vi "Expt4_MT PSK Transceiver_Student_lab.vi"(0 "Message Symbols":i32=1000, 5 "Eb/N0, dB":dbl(slide)=40.0 scale=0.0..80.0, 7 "TX Filter":T1(ring)=enum."Root Raised Cos", 9 "Reset":bool=TRUE, 14 "?":T2(tab)=enum."Constellation (RX output)") -> (3 "PSK System Parameters":T5={"samples per symbol (16)"=4, "symbol map"=[0.7071067811865476+0.7071067811865475i, -0.7071067811865475+0.7071067811865476i, 0.7071067811865474-0.7071067811865477i, -0.7071067811865477-0.7071067811865475i], "differential PSK"=enum."disable", "PSK type"=0} {"PSK type" items=["normal", "shifted", "offset"]; "symbol map" format="%.3f"}, 4 "Output Complex Waveform":cluster{"t0":dbl, "dt":dbl, "Values":cdb[]} {"Values" format="%.3f"; "dt" format="%^.2e"; "t0" format="%.4f"}, 6 "Transmitted  Bits":i8[](array[numeric]), 8 "Received Bits":i8[](array[numeric]), 10 "Bit Error Rate":dbl format="%.4e", 13 "Last Sync Found Index":dbl format="%.4f", 15 "Error Out":errorcluster)   [LabVIEW 2020]
doc: "This example demonstrates generation and analysis of PSK modulated signals. You can specify transmit filter parameters, Eb/No, and frequency offset. This example demonstrates programming techniques for resetting the transmitter in cases where the receiver (demodulator) lock is lost. You can see the results of the demodulation on an eye-diagram plot, and perform measurements such as bit error rate."
uses:
  <vilib>/addons/Modulation/niDMT.lvlib
  <vilib>/addons/Modulation/Digital/General/MT Format Eye Diagram (complex).vi
  <vilib>/addons/Modulation/niAMT.lvlib
  <vilib>/addons/Modulation/Digital/Support/Controls/PSK System Parameters.ctl
panel:
  out "Estimated Eb/N0(dB)":dbl
  out "Frequency Offset, Hz":dbl=0.0014081098665354938 format="%.2f"
  in  "Frequency Offset, Hz":dbl(slide) scale=-1000.0..1000.0
  in  "Symbol Rate":dbl=100000.0 step=1000.0 format="%.2p"
  in  "M-PSK":enum16{"2", "4", "8", "16", "32", "64"}(ring)=enum."4"
  out "Modulation Error Ratio, dB":dbl format="%.2f"
  out "BER Trigger Found":bool
  in  "Stop":bool
  out "TX Symbols":T3(graph)={{"1/x"=0.0, 1e-05, [], 1}, []}
  out "FFT Magnitude Spectrum":cluster{dbl, dbl, dbl[]}(graph)={-199899.99999999997, 99.99999999999999, []}
  out "Constellation graph":T4(graph)
  out "RX Symbols":T3(graph)={{"1/x"=0.0, 1e-05, [], 1}, []}
  in  "autoscale":bool
  out "Constellation Graph":T4(graph)
  in  "Display I/Q":enum16{"I", "Q"}(ring)=enum."Q"
  out "Eye Diagram":cluster{"t0":dbl, "dt":dbl, "Y":dbl[]}[](graph)
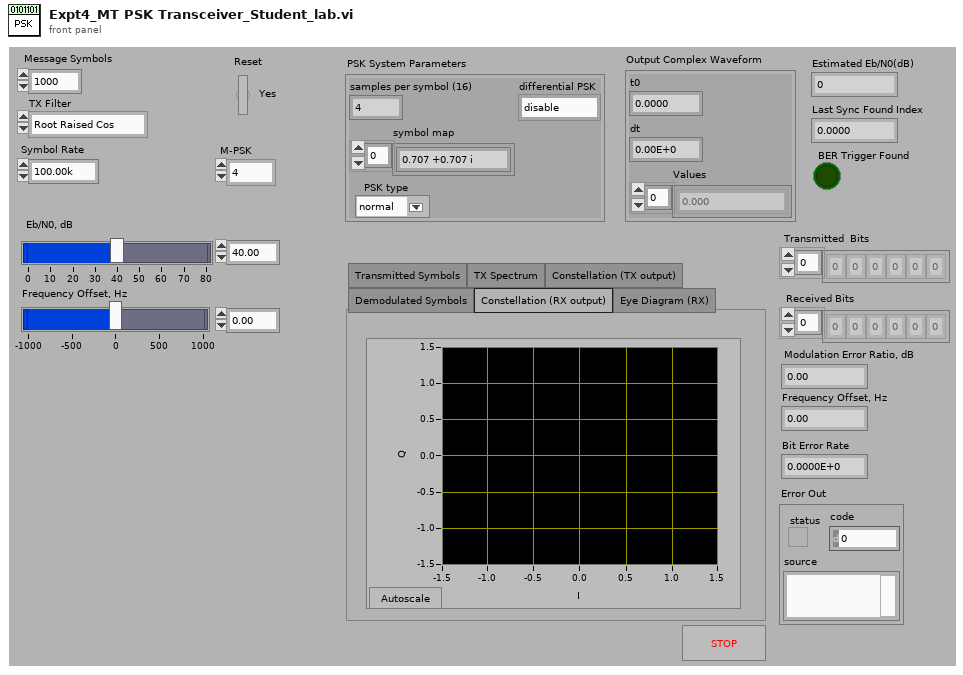
[diagram p1: front panel]
types:
  T1 = enum16{"none", "Raised Cosine", "Root Raised Cos", "Gaussian"}
  T2 = enum32{"Transmitted Symbols", "TX Spectrum", "Constellation (TX output)", "Demodulated Symbols", "Constellation (RX output)", "Eye Diagram (RX)"}
  T3 = cluster{cluster{"1/x":dbl, dbl, i8[], i32}, i32[][]}
  T4 = cluster{"Decimated Array":dbl[], "Decimated Array":dbl[]}[]
  T5 = typedef "niDMT.lvlib/PSK System Parameters.ctl" = cluster{"samples per symbol (16)":i32, "symbol map":cdb[], "differential PSK":enum16{"disable", "enable"}, "PSK type":u16}
  T6 = cluster{"expected sync location (symbols)":i32, "sync sequence":cdb[], "sync location uncertainty (symbols)":i32, "sync indent (symbols)":i32}
  T7 = cluster{"TX Filter":enum16{"none", "Raised Cosine", "Root Raised Cos", "Gaussian"}, "filter parameter":dbl, "filter length":i32}
  T8 = cluster{"M-PSK (4)":i32, "differential PSK":enum16{"disable", "enable"}, "PSK type":u16}
  T9 = cluster{"# Guard Bits":i32, "# Sync Bits":i32, "# Message Bits":i32, "PN sequence order":i32}
  T10 = cluster{"constellation":dbl[], "oversampled data":dbl[]}[]
  T11 = typedef "niAMT.lvlib/Complex Data Waveform.ctl" = cluster{"t0":dbl, "dt":dbl, "Y":cdb[]}
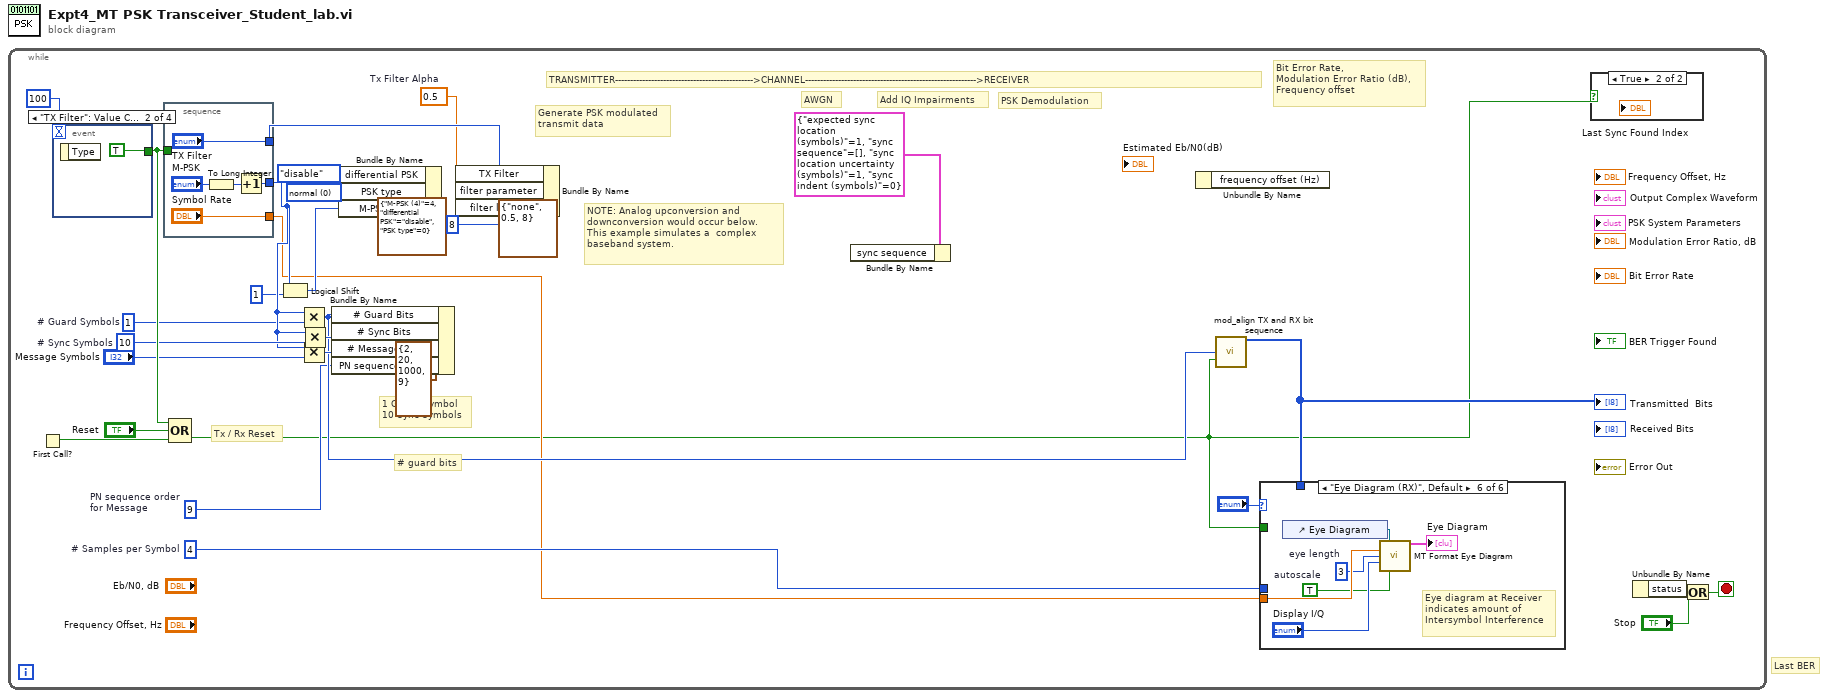
[diagram p0: block diagram]
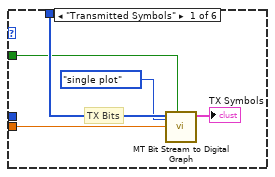
[diagram p2: hidden frame]
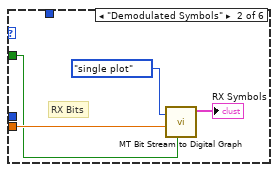
[diagram p3: hidden frame]
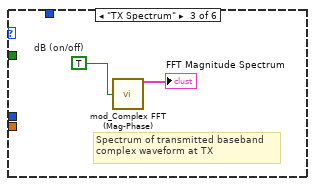
[diagram p4: hidden frame]
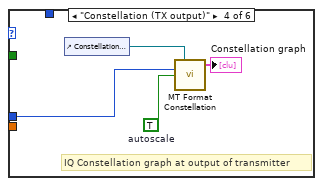
[diagram p5: hidden frame]
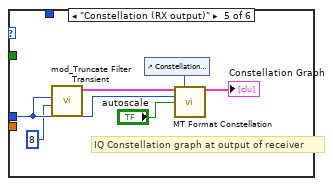
[diagram p6: hidden frame]
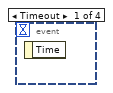
[diagram p8: hidden frame]
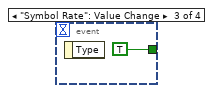
[diagram p9: hidden frame]
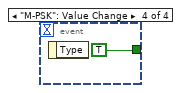
[diagram p10: hidden frame]
diagram:
  # "Last BER"
  n1 = while {
    stop <- w13 stop-if-true
    w3 = 9  # PN sequence order for Message
    w5 = 0.5  # Tx Filter Alpha
    w7 = u16 0 items=["normal", "shifted", "offset"] ("PSK type")
    w20 = 4  # # Samples per Symbol
    w23 = 10  # # Sync Symbols
    w16 = 1  # # Guard Symbols
    # "Bit Error Rate,\nModulation Error Ratio (dB),\nFrequency offset"
    # "Tx / Rx Reset"
    # "1 Guard Symbol\n10 Sync Symbols"
    # "# guard bits"
    # "Generate PSK modulated\ntransmit data"
    # "PSK Demodulation"
    # "Add IQ Impairments"
    # "AWGN"
    # "TRANSMITTER---------------------------------------------->CHANNEL--------------------------------------------------------->RECEIVER"
    # "NOTE: Analog upconversion and\ndownconversion would occur below.\nThis example simulates a  complex \nbaseband system."
    n2 = First Call?() -> (First Call?: T/F=w28:bool)
    n3 = event shown="[1] \"TX Filter\": Value Change" {
      selector: _ -> [_ _ _ _]
      dyn-events: _ -> [_ _ _ _]
      timeout: 100 -> [_ _ _ _]
      tunnel: [_ TRUE TRUE TRUE] -> w25
      event Timeout {
        n4 = event-data() -> ()  [unwired: 1 in, 1 out]
      }
      event "TX Filter": Value Change {
        n5 = event-data() -> ()  [unwired: 1 in, 1 out]
      }
      event "Symbol Rate": Value Change {
        n6 = event-data() -> ()  [unwired: 1 in, 1 out]
      }
      event "M-PSK": Value Change {
        n7 = event-data() -> ()  [unwired: 1 in, 1 out]
      }
    }
    n8 = stacked-sequence {
      tunnel: w25 -> [_]
      tunnel: ["TX Filter"] -> w21
      tunnel: [w32] -> w17
      tunnel: ["Symbol Rate"] -> w10
      frame #0 {
        n9 = To Long Integer(number="M-PSK") -> (32bit integer=w34:i32)
        n10 = Increment(x=w34) -> (x+1=w32:i32)
      }
    }
    n11 = Compound Arithmetic op=OR(w25, "Reset", w28) -> (w2:bool)
    n12 = Logical Shift(y=w17, x=1) -> (x << y=w12:i32)
    n13 = Multiply(x=w17, y=w16) -> (x*y=w15:i32)
    n14 = Multiply(x=w17, y="Message Symbols") -> (x*y=w18:i32)
    n15 = Multiply(x=w17, y=w23) -> (x*y=w22:i32)
    n16 = Bundle By Name(cluster=T9 {"# Guard Bits"=2, "# Sync Bits"=20, "# Message Bits"=1000, "PN sequence order"=9} ("Message"), "# Guard Bits"=w15, "# Sync Bits"=w22, "# Message Bits"=w18, "PN sequence order"=w3) -> ()  [unwired: 1 out]
    n17 = Bundle By Name(cluster=T8 {"M-PSK (4)"=4, "differential PSK"=enum."disable", "PSK type"=0} ("PSK"), "differential PSK"=enum16{"disable", "enable"}."disable", "PSK type"=w7, "M-PSK (4)"=w12) -> ()  [unwired: 1 out]
    n18 = Bundle By Name(cluster=T7 {"TX Filter"=enum."none", "filter parameter"=0.5, "filter length"=8} ("System Filter"), "TX Filter"=w21, "filter parameter"=w5, "filter length"=8) -> ()  [unwired: 1 out]
    n19 = Bundle By Name(cluster=T6 {"expected sync location (symbols)"=1, "sync sequence"=[], "sync location uncertainty (symbols)"=1, "sync indent (symbols)"=0} ("synchronization parameters")) -> ()  [unwired: 1 in, 1 out]
    n20 = Unbundle By Name() -> ()  [unwired: 1 in, 1 out]
    n21 = call <vilib>:"mod_align TX and RX bit sequence.vi"("# Bits removed"=w15, "Reset"=w2) -> ("Aligned array"=w14:i8[])  [unwired: 13 in]
    "Transmitted  Bits" <- w14
    n22 = case shown="\"Eye Diagram (RX)\", Default" "?" {
      tunnel: w10 -> [w40 w44 _ _ _ w62]
      tunnel: w20 -> [_ _ _ w47 w53 _]
      tunnel: w14 -> [w39 _ _ _ _ _]
      tunnel: w2 -> [w38 w41 _ _ _ _]
      frame "Transmitted Symbols" {
        # "TX Bits"
        n23 = call <vilib>:"MT Bit Stream to Digital Graph.vi"("Reset (F)"=w38, "Format"=enum16{"single plot", "plot per bit"}."single plot", "Symbol Rate (Hz)"=w40, "Bit Stream"=w39) -> ("Digital Waveform Graph"=→"TX Symbols":T3)  [unwired: 7 in]
      }
      frame "Demodulated Symbols" {
        # "RX Bits"
        n24 = call <vilib>:"MT Bit Stream to Digital Graph.vi"("Reset (F)"=w41, "Format"=enum16{"single plot", "plot per bit"}."single plot", "Symbol Rate (Hz)"=w44) -> ("Digital Waveform Graph"=→"RX Symbols":T3)  [unwired: 8 in]
      }
      frame "TX Spectrum" {
        w45 = TRUE  # dB (on/off)
        # "Spectrum of transmitted baseband\ncomplex waveform at TX"
        n25 = call <vilib>:"mod_Complex FFT (Mag-Phase).vi"("dB (on/off)"=w45) -> ("Magnitude"=→"FFT Magnitude Spectrum":cluster{"f0":dbl, "df":dbl, "Y":dbl[]})  [unwired: 13 in, 1 out]
      }
      frame "Constellation (TX output)" {
        w50 = TRUE  # autoscale
        # "IQ Constellation graph at output of transmitter"
        n26 = control-ref of="Constellation graph"() -> (w48:refnum<vi>)
        n27 = call <vilib>:"MT Format Constellation.vi"("constellation reference"=w48, "samples per symbol"=w47, "autoscale"=w50) -> ("constellation graph"=→"Constellation graph":T10)  [unwired: 11 in, 1 out]
      }
      frame "Constellation (RX output)" {
        # "IQ Constellation graph at output of receiver"
        n28 = call <vilib>:"mod_Truncate Filter Transient.vi"("filter length (sym)"=8, "samples/symbol"=w53) -> ("output complex waveform"=w54:T11)  [unwired: 9 in]
        n29 = control-ref of="Constellation Graph"() -> (w55:refnum<vi>)
        n30 = call <vilib>:"MT Format Constellation.vi"("waveform"=w54, "constellation reference"=w55, "samples per symbol"=w53, "autoscale"="autoscale") -> ("constellation graph"=→"Constellation Graph":T10)  [unwired: 10 in, 1 out]
      }
      frame "Eye Diagram (RX)", Default {
        w59 = TRUE  # autoscale
        w61 = 3  # eye length
        # "Eye diagram at Receiver\nindicates amount of\nIntersymbol Interference"
        n31 = control-ref of="Eye Diagram"() -> (w57:refnum<vi>)
        n32 = call-poly <vilib>:"MT Format Eye Diagram.vi"("eye diagram reference"=w57, "symbol rate (Hz)"=w62, "eye length"=w61, "I/Q (I)"="Display I/Q", "autoscale"=w59) -> ("eye diagram"=→"Eye Diagram":cluster{"t0":dbl, "dt":dbl, "Y":dbl[]}[])  [unwired: 9 in, 1 out]
      }
    }
    n33 = case shown="True" w2 {
      frame False {
      }
      frame True {
      }
    }
    n34 = Unbundle By Name() -> ()  [unwired: 1 in, 1 out]
    n35 = Or(y="Stop") -> (x .or. y?=w13:bool)  [unwired: 1 in]
  }
